vi "GamePiecePose2.vi"(0 "GamePiece Valid [t-?]":bool, 1 "Robot Heading (deg)":dbl, 2 "Odometry Timestamp (ms)":u32, 3 "GamePiece Timestamp (ms)":u32, 5 "GamePiece Type [t-?]":enum16{"None", "Cube", "Cone"}(ring), 7 "Y (in) [t0]":dbl, 9 "X (in) [t0]":dbl, 12 "GamePiece Ty (deg) [t-?]":dbl, 13 "GamePiece Tx (deg) [t-?]":dbl) -> (4 "GamePiece Y (in) [t-?]":dbl, 6 "GamePiece X (in) [t-?]":dbl, 8 "GamePiece Valid [t-?]":bool, 10 "GamePiece Range (in) [t-?":dbl)   [LabVIEW 2020]
doc: "Calculates the detected game piece pose relative to the robot using data from the LimeLight camera. Also performs additional validation checks to determine if the game piece vision data should be trusted."
uses:
  54abcb88-3220-419e-9bec-4c3c6f5e2905.vi
  76103391-ba62-4dc0-bcc0-26de5557a5b7.vi
  e823d307-d35b-45d7-a729-51121ade1bdb.vi
  4f3d002f-ad2c-48f1-81b6-0e59c3cd0741.vi
  GlobalPoseAndTargeting.vi
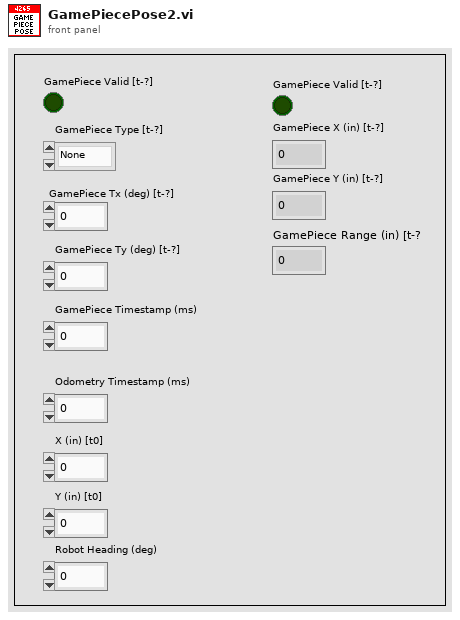
[diagram p1: front panel]
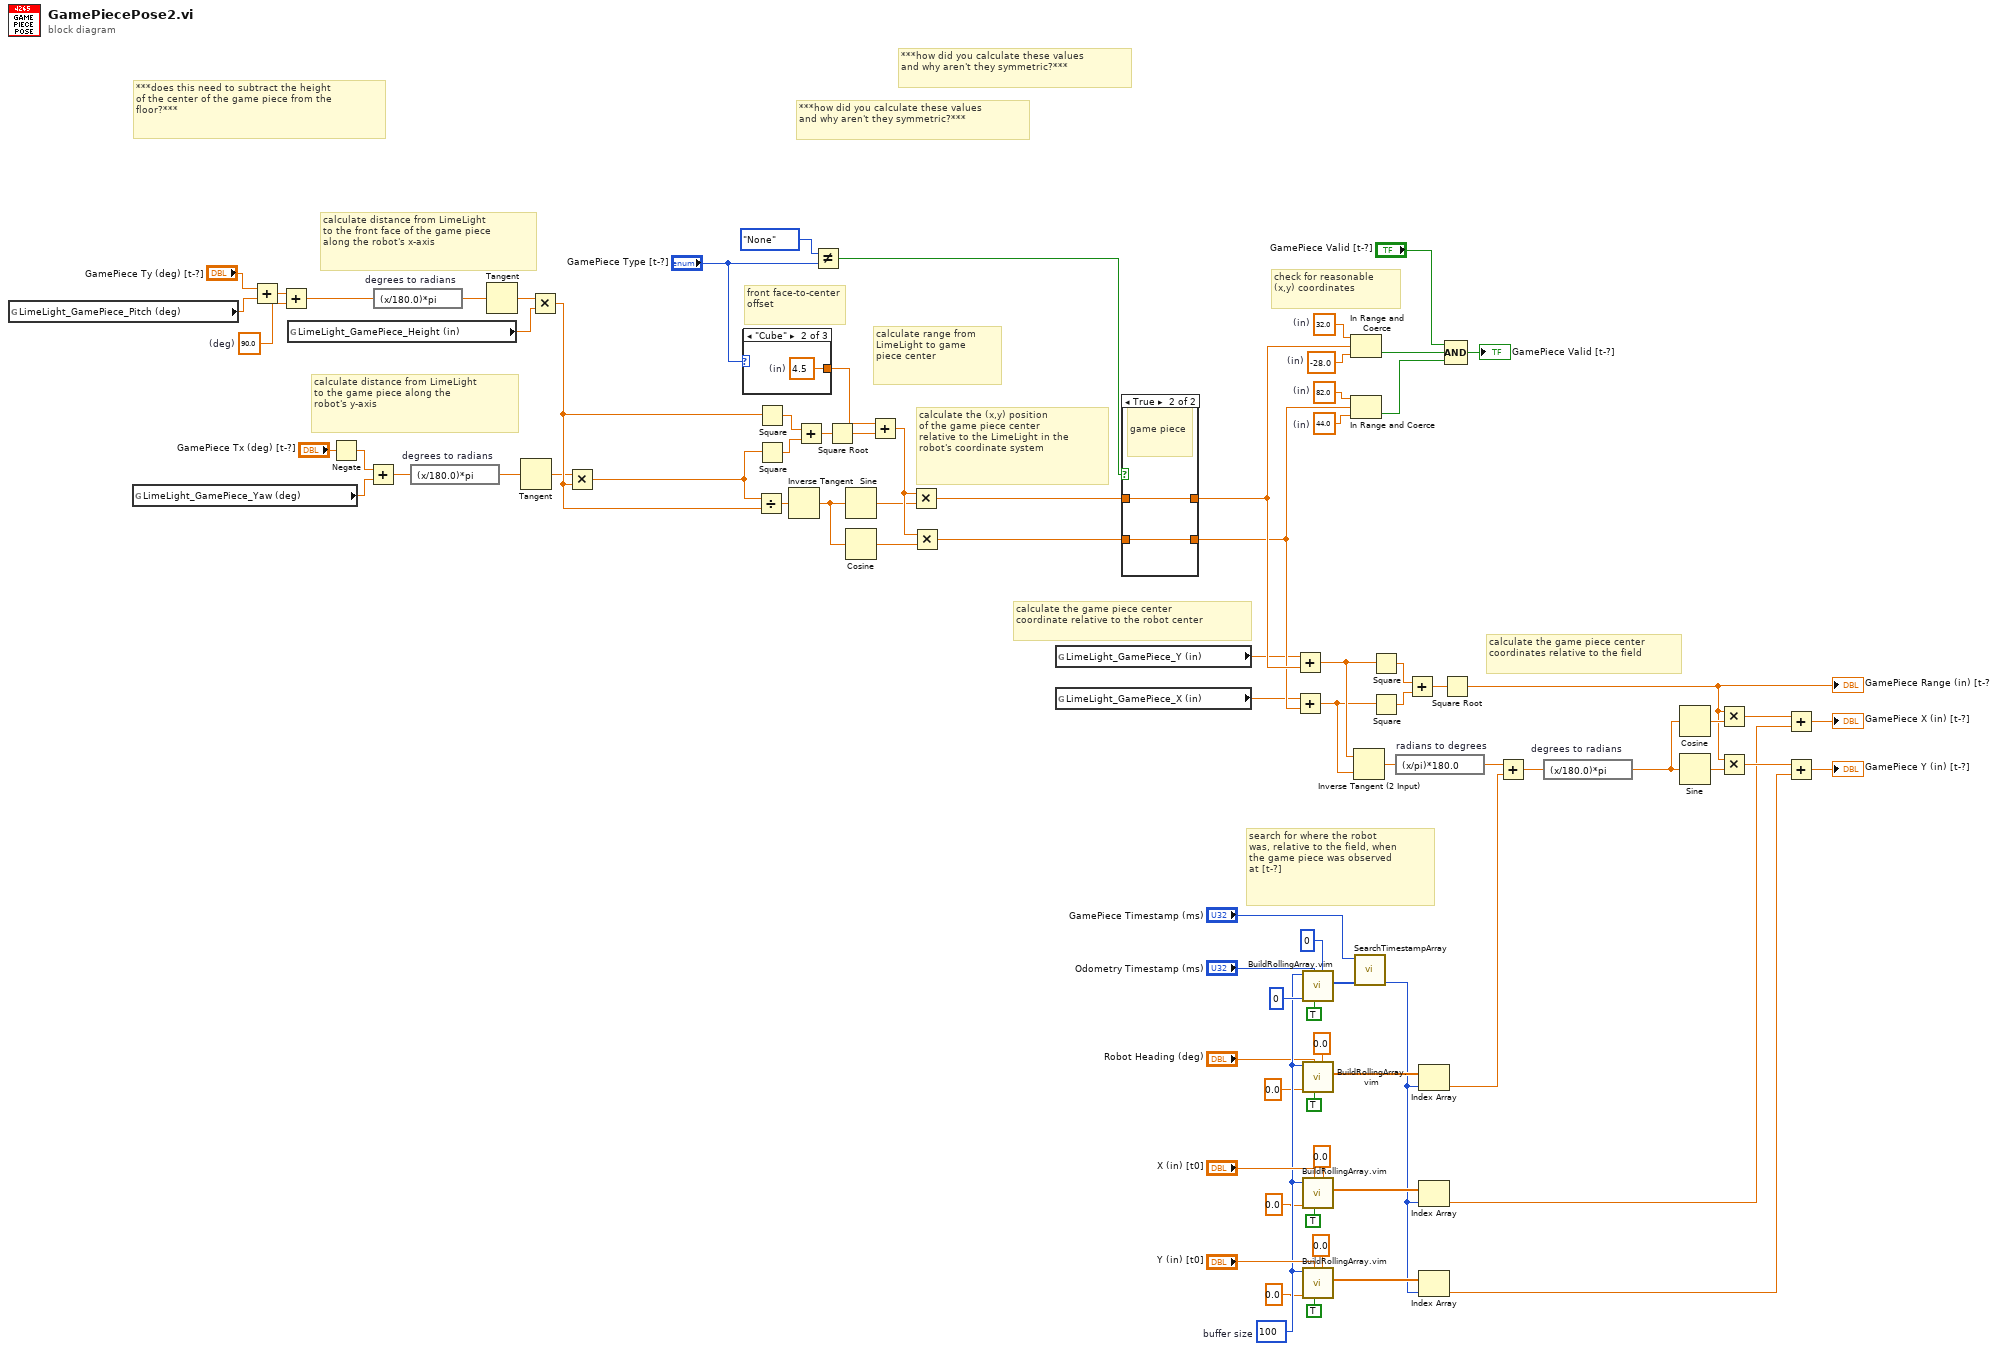
[diagram p0: block diagram]
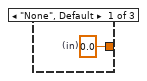
[diagram p2: hidden frame]
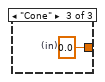
[diagram p3: hidden frame]
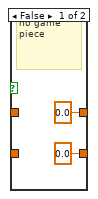
[diagram p4: hidden frame]
diagram:
  w32 = 100  # buffer size
  w57 = 44.0  # (in)
  w58 = 82.0  # (in)
  w59 = -28.0  # (in)
  w60 = 32.0  # (in)
  w72 = 90.0  # (deg)
  # "***how did you calculate these values\nand why aren't they symmetric?***"
  # "***how did you calculate these values\nand why aren't they symmetric?***"
  # "search for where the robot\nwas, relative to the field, when\nthe game piece was observed\nat [t-?]"
  # "calculate the game piece center\ncoordinates relative to the field"
  # "check for reasonable\n(x,y) coordinates"
  # "calculate the game piece center\ncoordinate relative to the robot center"
  # "***does this need to subtract the height\nof the center of the game piece from the\nfloor?***"
  # "calculate the (x,y) position\nof the game piece center \nrelative to the LimeLight in the\nrobot's coordinate system"
  # "calculate range from\nLimeLight to game\npiece center"
  # "calculate distance from LimeLight\nto the game piece along the\nrobot's y-axis"
  # "calculate distance from LimeLight\nto the front face of the game piece\nalong the robot's x-axis"
  # "front face-to-center offset"
  n1 = global read "GlobalPoseAndTargeting.vi" "LimeLight_GamePiece_Pitch (deg)"() -> (w16:dbl)
  n2 = global read "GlobalPoseAndTargeting.vi" "LimeLight_GamePiece_Yaw (deg)"() -> (w66:dbl)
  n3 = Add(x="GamePiece Ty (deg) [t-?]", y=w16) -> (x+y=w21:dbl)
  n4 = Add(x=w21, y=w72) -> (x+y=w71:dbl)
  n5 = global read "GlobalPoseAndTargeting.vi" "LimeLight_GamePiece_Height (in)"() -> (w20:dbl)
  n6 = Negate(x="GamePiece Tx (deg) [t-?]") -> (-x=w54:dbl)
  n7 = Add(x=w54, y=w66) -> (x+y=w73:dbl)
  n8 = expression code="(x/180.0)*pi" "degrees to radians"(w71) -> (w70:dbl)
  n9 = expression code="(x/180.0)*pi" "degrees to radians"(w73) -> (w74:dbl)
  n10 = Tangent(1:w70) -> (0:w69:dbl)
  n11 = Tangent(1:w74) -> (0:w75:dbl)
  n12 = Multiply(x=w69, y=w20) -> (x*y=w81:dbl)
  n13 = Multiply(x=w75, y=w81) -> (x*y=w82:dbl)
  n14 = case shown="\"Cube\"" "GamePiece Type [t-?]" {
    tunnel: [w86 w87 w88] -> w10
    frame "None", Default {
      w86 = 0.0  # (in)
    }
    frame "Cube" {
      w87 = 4.5  # (in)
    }
    frame "Cone" {
      w88 = 0.0  # (in)
    }
  }
  n15 = Divide(x=w82, y=w81) -> (x/y=w77:dbl)
  n16 = Square(x=w81) -> (x^2=w12:dbl)
  n17 = Square(x=w82) -> (x^2=w11:dbl)
  n18 = Inverse Tangent(1:w77) -> (0:w79:dbl)
  n19 = Add(x=w12, y=w11) -> (x+y=w76:dbl)
  n20 = Not Equal?(x=enum16{"None", "Cube", "Cone"}."None" ("y"), y="GamePiece Type [t-?]") -> (x != y?=w68:bool)
  n21 = Square Root(x=w76) -> (sqrt(x)=w9:dbl)
  n22 = Sine(x=w79) -> (sin(x)=w78:dbl)
  n23 = Cosine(x=w79) -> (cos(x)=w80:dbl)
  n24 = Add(x=w10, y=w9) -> (x+y=w83:dbl)
  n25 = Multiply(x=w83, y=w78) -> (x*y=w84:dbl)
  n26 = Multiply(x=w83, y=w80) -> (x*y=w85:dbl)
  n27 = global read "GlobalPoseAndTargeting.vi" "LimeLight_GamePiece_Y (in)"() -> (w56:dbl)
  n28 = global read "GlobalPoseAndTargeting.vi" "LimeLight_GamePiece_X (in)"() -> (w55:dbl)
  n29 = case shown="True" w68 {
    tunnel: w84 -> [_ w92]
    tunnel: [0.0 w92] -> w65
    tunnel: w85 -> [_ w91]
    tunnel: [0.0 w91] -> w64
    frame False {
      # "no game piece"
    }
    frame True {
      # "game piece"
    }
  }
  n30 = Add(x=w56, y=w65) -> (x+y=w19:dbl)
  n31 = Add(x=w55, y=w64) -> (x+y=w18:dbl)
  n32 = call "BuildRollingArray.vim"("Global Additive Update"=0, "Update?"=TRUE, "New Value"="Odometry Timestamp (ms)", "Initial Value"=0, "Number of Elements"=w32) -> ("Current Array"=w44:u32[])  [unwired: 6 in]
  n33 = call "BuildRollingArray.vim"("Global Additive Update"=0.0, "Update?"=TRUE, "New Value"="Robot Heading (deg)", "Initial Value"=0.0, "Number of Elements"=w32) -> ("Current Array"=w34:dbl[])  [unwired: 6 in]
  n34 = call "BuildRollingArray.vim"("Global Additive Update"=0.0, "Update?"=TRUE, "New Value"="X (in) [t0]", "Initial Value"=0.0, "Number of Elements"=w32) -> ("Current Array"=w43:dbl[])  [unwired: 6 in]
  n35 = call "BuildRollingArray.vim"("Global Additive Update"=0.0, "Update?"=TRUE, "New Value"="Y (in) [t0]", "Initial Value"=0.0, "Number of Elements"=w32) -> ("Current Array"=w42:dbl[])  [unwired: 6 in]
  n36 = In Range and Coerce(upper limit=w60, x=w65, lower limit=w59) -> (In Range?=w62:bool)  [unwired: 1 out]
  n37 = In Range and Coerce(upper limit=w58, x=w64, lower limit=w57) -> (In Range?=w61:bool)  [unwired: 1 out]
  n38 = Inverse Tangent (2 Input)(1:w18, 2:w19) -> (0:w14:dbl)
  n39 = call "SearchTimestampArray.vi"("Timestamp Array"=w44, "Search Timestamp"="GamePiece Timestamp (ms)") -> ("Closest Index"=w33:i32)  [unwired: 8 in, 1 out]
  n40 = Square(x=w19) -> (x^2=w48:dbl)
  n41 = Square(x=w18) -> (x^2=w49:dbl)
  n42 = expression code="(x/pi)*180.0" "radians to degrees"(w14) -> (w13:dbl)
  n43 = Add(x=w48, y=w49) -> (x+y=w50:dbl)
  n44 = Index Array(array=w34, index=w33) -> (element=w30:dbl)
  n45 = Index Array(array=w43, index=w33) -> (element=w23:dbl)
  n46 = Index Array(array=w42, index=w33) -> (element=w22:dbl)
  n47 = Square Root(x=w50) -> (sqrt(x)=w15:dbl)
  "GamePiece Range (in) [t-?" <- w15
  n48 = Compound Arithmetic op=AND("GamePiece Valid [t-?]", w62, w61) -> (→"GamePiece Valid [t-?]":bool)
  n49 = Add(x=w13, y=w30) -> (x+y=w47:dbl)
  n50 = expression code="(x/180.0)*pi" "degrees to radians"(w47) -> (w51:dbl)
  n51 = Cosine(x=w51) -> (cos(x)=w52:dbl)
  n52 = Sine(x=w51) -> (sin(x)=w53:dbl)
  n53 = Multiply(x=w15, y=w52) -> (x*y=w24:dbl)
  n54 = Multiply(x=w15, y=w53) -> (x*y=w25:dbl)
  n55 = Add(x=w24, y=w23) -> (x+y=→"GamePiece X (in) [t-?]":dbl)
  n56 = Add(x=w25, y=w22) -> (x+y=→"GamePiece Y (in) [t-?]":dbl)
